vi "Convert-speed.vi"(8 "error in (no error)":errorcluster, 10 "Speed in":dbl caption="Speed [unit/s]", 11 "Motor in":refnum<class "Motor.lvclass">) -> (0 "error out":errorcluster, 2 "Speed out":dbl caption="Speed out [rpm]", 3 "Motor out":refnum<class "Motor.lvclass">)   [LabVIEW 2013, in "PowderDeposition.lvlib" / "Motor.lvclass"]
uses:
  Motor.lvclass
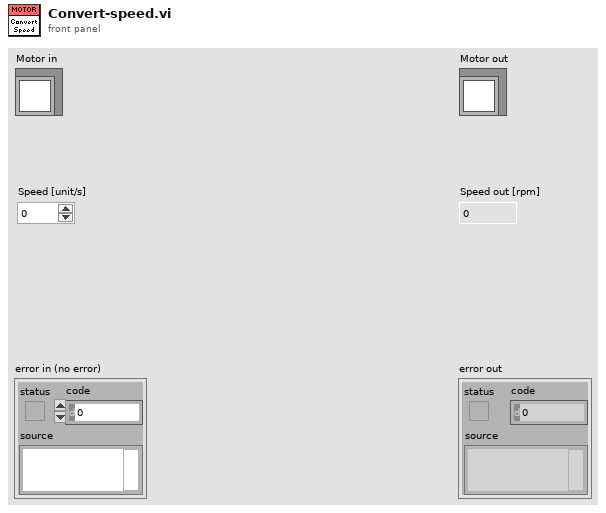
[diagram p1: front panel]
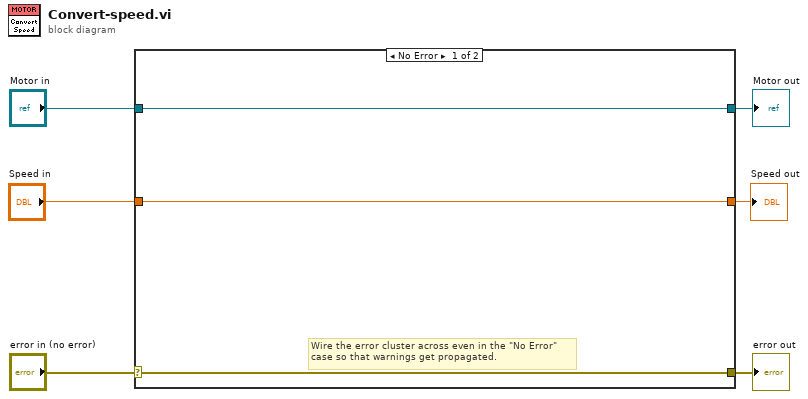
[diagram p0: block diagram]
diagram:
  n1 = case shown="No Error" "error in (no error)" {
    selector: "error in (no error)" -> [w7 w12]
    tunnel: [w7 w12] -> w5
    tunnel: [w8 w11] -> w3
    tunnel: "Motor in" -> [w8 w11]
    tunnel: "Speed in" -> [w9 w10]
    tunnel: [w9 w10] -> w1
    frame No Error {
      # "Wire the error cluster across even in the \"No Error\"\ncase so that warnings get propagated."
    }
    frame Error {
    }
  }
  "error out" <- w5
  "Motor out" <- w3
  "Speed out" <- w1
